vi "Show Front Panel (private).vi"(8 "Error In":errorcluster, 11 "VI Reference":refnum<vi>) -> (0 "Error Out":errorcluster)   [LabVIEW 2023, in "Error Manager.lvlib"]
doc: "This VI configures the Front Panel (the GUI) of the Error Manager VI. This VI is expected to be called when the user presses an \"Error\" button to view the list of errors."
uses:
  Error Manager.lvlib
  <vilib>/Utility/miscctls.llb/LVPointTypeDef.ctl
  <vilib>/Utility/miscctls.llb/LVRectTypeDef.ctl
panel:
  # "Development\ncontrols/indicators useful for development and testing, but which are not outputs of the VI"
  # "Input\nInputs to the VI"
  # "Output\nOutputs of the VI"
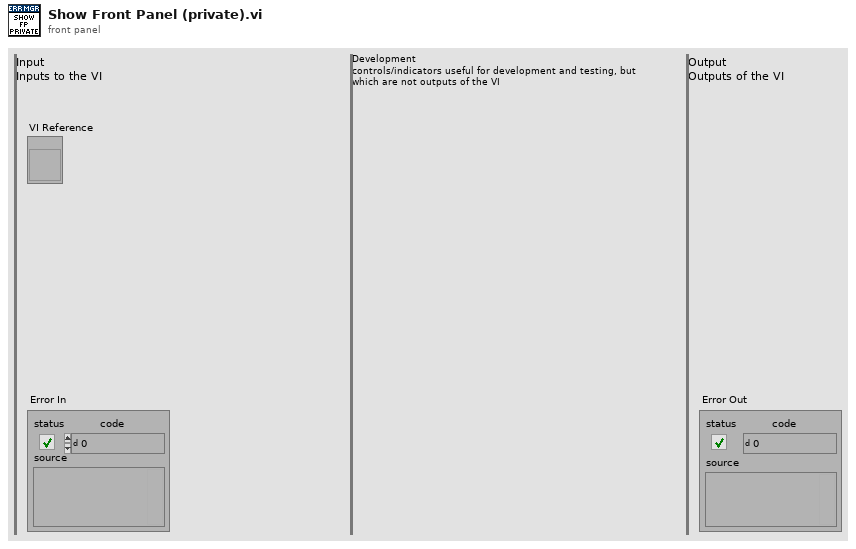
[diagram p1: front panel]
types:
  T1 = typedef "LVRectTypeDef.ctl" = cluster{"Left":i16, "Top":i16, "Right":i16, "Bottom":i16}
  T2 = typedef "LVPointTypeDef.ctl" = cluster{"Horizontal":i16, "Vertical":i16}
  T3 = enum32{"Invalid", "Default", "Floating", "Floating/Auto-Hide", "Modal"}
  T4 = enum32{"Invalid", "Standard", "Closed", "Hidden", "Minimized", "Maximized"}
  T5 = enum16{"Always On", "Always Off", "Off While Running"}
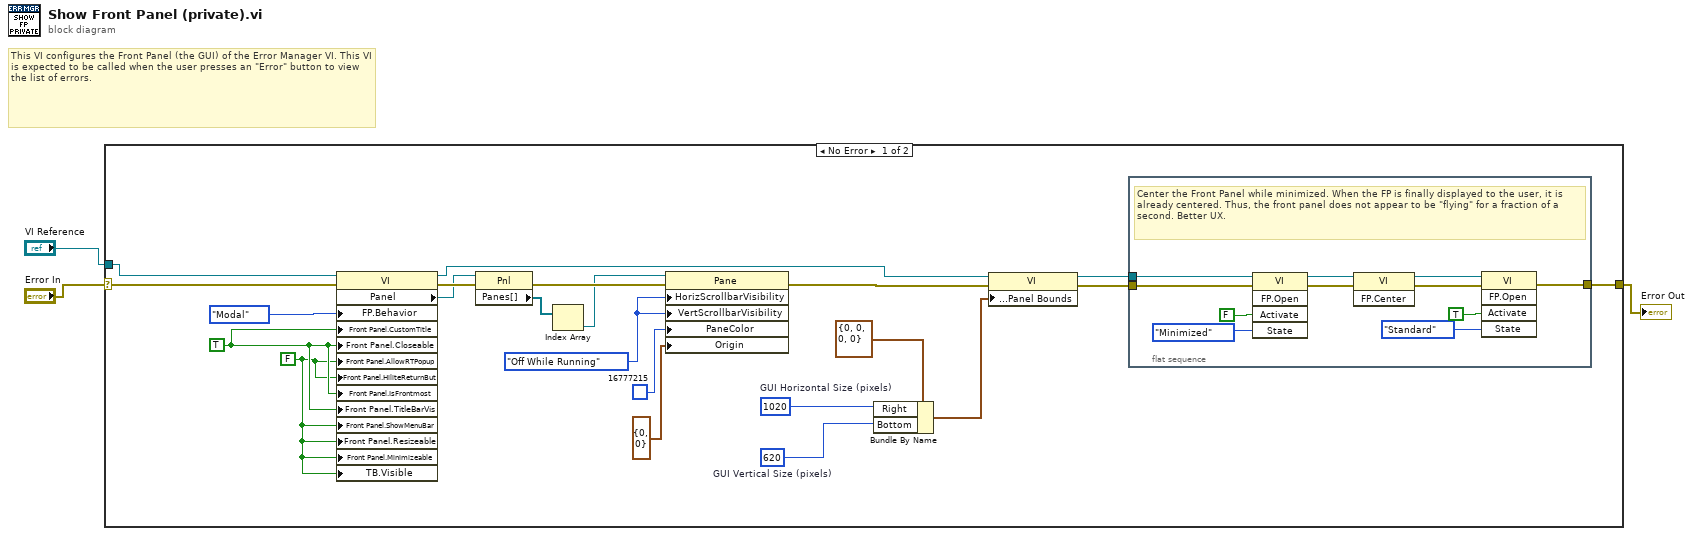
[diagram p0: block diagram]
diagram:
  # "This VI configures the Front Panel (the GUI) of the Error Manager VI. This VI is expected to be called when the user presses an \"Error\" button to view the list of errors."
  n1 = case shown="No Error" "Error In" {
    selector: "Error In" -> [w25 w37]
    tunnel: [w13 w37] -> w1
    tunnel: "VI Reference" -> [w23 _]
    frame No Error {
      w5 = i16 620  # GUI Vertical Size (pixels)
      w6 = i16 1020  # GUI Horizontal Size (pixels)
      w16 = T5."Off While Running" ("Horizontal Scrollbar Visibility")
      w14 = FALSE
      w21 = TRUE
      n2 = property class="VI"(reference=w23, error in=w25, "FP.Behavior"=T3."Modal" ("Front Panel Window:Behavior"), "Front Panel.CustomTitle"=w21, "Front Panel.Closeable"=w21, "Front Panel.AllowRTPopup"=w14, "Front Panel.HiliteReturnBut"=w14, "Front Panel.IsFrontmost"=w21, "Front Panel.TitleBarVis"=w21, "Front Panel.ShowMenuBar"=w14, "Front Panel.Resizeable"=w14, "Front Panel.Minimizeable"=w14, "TB.Visible"=w14) -> (reference out=w9:refnum<vi>, error out=w24:errorcluster, "Panel"=w19:refnum<vi>)
      n3 = property class="Pnl"(reference=w19, error in=w24) -> (error out=w20:errorcluster, "Panes[]"=w18:refnum<vi>[])  [unwired: 1 out]
      n4 = Index Array(array=w18) -> (element=w17:refnum<vi>)  [unwired: 1 in]
      n5 = property class="Pane"(reference=w17, error in=w20, "HorizScrollbarVisibility"=w16, "VertScrollbarVisibility"=w16, "PaneColor"=u32 16777215, "Origin"=T2 {"Horizontal"=0, "Vertical"=0}) -> (error out=w11:errorcluster)  [unwired: 1 out]
      n6 = Bundle By Name(cluster=T1 {"Left"=0, "Top"=0, "Right"=0, "Bottom"=0} ("Front Panel Window:Panel Bounds"), "Right"=w6, "Bottom"=w5) -> (w7:T1)
      n7 = property on="Property Node" class="VI"(reference=w9, error in=w11, "Front Panel Window:Panel Bounds"=w7) -> (reference out=w4:refnum<vi>, error out=w10:errorcluster)
      n8 = flat-sequence {
        tunnel: [w36] -> w13
        tunnel: w10 -> [w33]
        tunnel: w4 -> [w29]
        frame #0 {
          # "Center the Front Panel while minimized. When the FP is finally displayed to the user, it is already centered. Thus, the front panel does not appear to be \"flying\" for a fraction of a second. Better UX."
          n9 = invoke class="VI" method="FP.Open"(reference=w29, error in=w33, "Activate"=FALSE ("Activate?"), "State"=T4."Minimized") -> (reference out=w28:refnum<vi>, error out=w30:errorcluster)  [unwired: 1 in, 3 out]
          n10 = invoke class="VI" method="FP.Center"(reference=w28, error in=w30) -> (reference out=w31:refnum<vi>, error out=w32:errorcluster)  [unwired: 1 in, 1 out]
          n11 = invoke class="VI" method="FP.Open"(reference=w31, error in=w32, "Activate"=TRUE ("Activate?"), "State"=T4."Standard") -> (error out=w36:errorcluster)  [unwired: 1 in, 4 out]
        }
      }
    }
    frame Error {
    }
  }
  "Error Out" <- w1
